vi "MyRIO_Main.vi"() -> ()   [LabVIEW 2019]
uses:
  <vilib>/myRIO/Instrument Drivers/Onboard IO/DIO/typedefs/DIO Reference.ctl
  <vilib>/myRIO/Common/Instrument Driver Framework/Utilities/typedefs/myRIO Generic Hardware Reference.ctl
  <vilib>/myRIO/Common/Instrument Driver Framework/Utilities/typedefs/Hardware Version Enum.ctl
  <vilib>/myRIO/Common/Instrument Driver Framework/Utilities/typedefs/myRIO v1.0 Reference.ctl
  <vilib>/myRIO/Common/Instrument Driver Framework/Utilities/typedefs/Generic FPGA Reference.ctl
  <vilib>/myRIO/Common/Instrument Driver Framework/myRIO v1.0/DIO/typedefs/DIO Channels List.ctl
  <vilib>/myRIO/Common/Instrument Driver Framework/myRIO v1.0/DIO/typedefs/DIO Channels Enum.ctl
  <vilib>/userDefined/High Color/nirio_resource_hc.ctl
  <vilib>/myRIO/Instrument Drivers/Onboard Devices/Accelerometer/typedefs/Accelerometer Reference.ctl
  <vilib>/myRIO/Common/Instrument Driver Framework/myRIO v1.0/Accelerometer/typedefs/Accelerometer Channels List.ctl
  <vilib>/myRIO/Common/Instrument Driver Framework/myRIO v1.0/Accelerometer/typedefs/Accelerometer Channels Enum.ctl
  <vilib>/myRIO/Common/Instrument Driver Framework/Utilities/vis/Is FPGA Ref Available.vi
  <vilib>/myRIO/Common/Instrument Driver Framework/myRIO v1.0/DIO/vis/myRIO v1.1 Open DIO.vi
  <vilib>/myRIO/Instrument Drivers/Onboard IO/DIO/vis/Read.vi
  <vilib>/myRIO/Common/Instrument Driver Framework/myRIO v1.0/Accelerometer/vis/myRIO v1.1 Open Accelerometer.vi
  <vilib>/myRIO/Instrument Drivers/Onboard Devices/Accelerometer/vis/Read.vi
  <vilib>/myRIO/Instrument Drivers/Onboard IO/DIO/vis/Write.vi
  <vilib>/myRIO/Common/Instrument Driver Framework/Utilities/vis/Validate Channels.vi
  <vilib>/myRIO/Common/Instrument Driver Framework/myRIO v1.0/DIO/vis/myRIO v1.0 Reserve DIO.vi
  <vilib>/myRIO/Common/Instrument Driver Framework/myRIO v1.0/Accelerometer/vis/myRIO v1.0 Reserve Accelerometer.vi
  <vilib>/myRIO/Common/Instrument Driver Framework/myRIO v1.0/Resource Manager/vis/myRIO v1.0 Reserve Channel List.vi
  <vilib>/myRIO/Common/Instrument Driver Framework/myRIO v1.0/DIO/vis/myRIO v1.0 Build MUX Configuration DIO.vi
  <vilib>/myRIO/Common/Instrument Driver Framework/myRIO v1.0/Accelerometer/vis/myRIO v1.0 Build MUX Configuration Accelerometer.vi
  <vilib>/myRIO/Common/Instrument Driver Framework/myRIO v1.0/Resource Manager/vis/myRIO v1.0 Reserve Channel.vi
  <vilib>/myRIO/Common/Instrument Driver Framework/myRIO v1.0/Resource Manager/vis/myRIO v1.0 Unreserve Channel.vi
  <vilib>/myRIO/Common/Instrument Driver Framework/myRIO v1.0/Resource Manager/vis/myRIO v1.0 Create Configuration List.vi
  <vilib>/myRIO/Common/Instrument Driver Framework/myRIO v1.0/Resource Manager/vis/myRIO v1.0 Build Mutex Name.vi
  <vilib>/Utility/VariantDataType/GetNumericInfo.vi
  <vilib>/Utility/error.llb/Error Cluster From Error Code.vi
  <vilib>/myRIO/Common/Instrument Driver Framework/myRIO v1.0/myRIO v1.1 Open.vi
  <vilib>/myRIO/Common/Instrument Driver Framework/Utilities/vis/IO Manager.vi
  <vilib>/myRIO/Common/Instrument Driver Framework/Utilities/vis/Configuration Manager.vi
  <vilib>/myRIO/Common/Instrument Driver Framework/myRIO v1.0/Resource Manager/vis/myRIO v1.0 Configure IO.vi
  <vilib>/myRIO/Common/Instrument Driver Framework/myRIO v1.0/myRIO v1.0 Close.vi
  <vilib>/myRIO/Common/Instrument Driver Framework/myRIO v1.0/DIO/vis/myRIO v1.0 Read DIO.vi
  <vilib>/myRIO/Common/Instrument Driver Framework/myRIO v1.0/Accelerometer/vis/myRIO v1.0 Get Scaling Constant Accelerometer.vi
  <vilib>/myRIO/Common/Instrument Driver Framework/myRIO v1.0/Accelerometer/vis/myRIO v1.0 Read Accelerometer.vi
  <vilib>/myRIO/Common/Instrument Driver Framework/myRIO v1.0/DIO/vis/myRIO v1.0 Write DIO.vi
  <vilib>/myRIO/Express VI/Onboard Devices/Button/Button Express VI.xnode
  <vilib>/myRIO/Instrument Drivers/Onboard IO/DIO/vis/myRIO DIO Open.xnode
  <vilib>/myRIO/Express VI/Onboard Devices/Accelerometer/Accelerometer Express VI.xnode
  <vilib>/myRIO/Instrument Drivers/Onboard Devices/Accelerometer/vis/myRIO Accelerometer Open.xnode
  <vilib>/myRIO/Express VI/Onboard Devices/LED/LED Express VI.xnode
  <vilib>/myRIO/Instrument Drivers/Onboard IO/DIO/DIO.lvlib
  <vilib>/myRIO/Instrument Drivers/Onboard Devices/Accelerometer/Accelerometer.lvlib
panel:
  out "angke":dbl
  out "z":dbl
  out "y":dbl
  in  "stop":bool
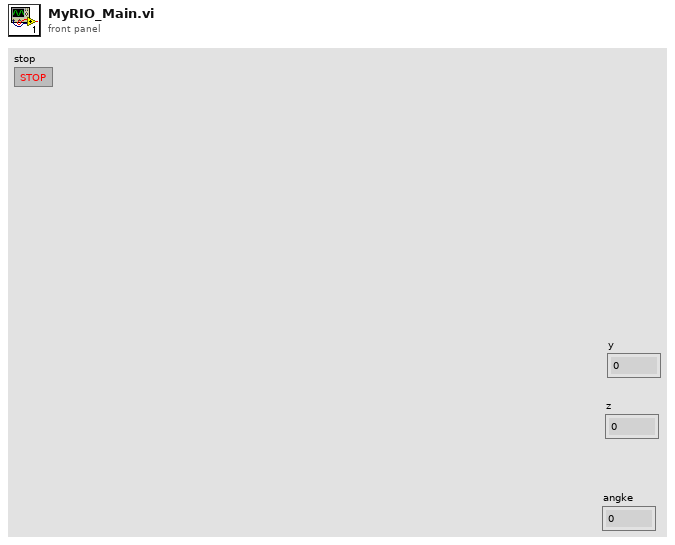
[diagram p1: front panel]
types:
  T1 = typedef "Accelerometer.lvlib/Accelerometer Reference.ctl" = cluster{"myRIO Reference":T2, "Accelerometer Channels List":T6, "LSB Weight":dbl}
  T2 = typedef "myRIO Generic Hardware Reference.ctl" = cluster{"myRIO Model":T3, "myRIO Hardware Reference":T4}
  T3 = typedef "Hardware Version Enum.ctl" = enum16{"Unknown", "myRIO-1900", "myRIO-1950", "roboRIO", "NI ELVIS RIO CM", "ELVIS III"}
  T4 = typedef "myRIO v1.0 Reference.ctl" = cluster{"Generic FPGA Reference":T5, "Allow multiple opens":bool}
  T5 = typedef "Generic FPGA Reference.ctl" = refnum<k20>
  T6 = typedef "Accelerometer Channels List.ctl" = T7[]
  T7 = typedef "Accelerometer Channels Enum.ctl" = enum16{"Not Connected", "X-Axis", "Y-Axis", "Z-Axis"}
  T8 = typedef "nirio_resource_hc.ctl" = tag
  T9 = typedef "DIO.lvlib/DIO Reference.ctl" = cluster{"myRIO Reference":T2, "DIO Channels List":T10}
  T10 = typedef "DIO Channels List.ctl" = T11[]
  T11 = typedef "DIO Channels Enum.ctl" = enum16{"Not Connected", "C/DIO0", "C/DIO1", "C/DIO2", "C/DIO3", "C/DIO4", "C/DIO5", "C/DIO6", "C/DIO7", "A/DIO0", "A/DIO1", "A/DIO2", "A/DIO3", "A/DIO4", "A/DIO5", "A/DIO6", "A/DIO7", "A/DIO8", "A/DIO9", "A/DIO10", "A/DIO11", "A/DIO12", "A/DIO13", "A/DIO14", "A/DIO15", "A/DIO16", "A/DIO17", "A/DIO18", "A/DIO19", "B/DIO0", "B/DIO1", "B/DIO2", "B/DIO3", "B/DIO4", "B/DIO5", "B/DIO6", "B/DIO7", "B/DIO8", "B/DIO9", "B/DIO10", "B/DIO11", "B/DIO12", "B/DIO13", "B/DIO14", "B/DIO15", "B/DIO16", "B/DIO17", "B/DIO18", "B/DIO19", "LED0", "LED1", "LED2", "LED3", "Button0", "DIO/DIO0", "DIO/DIO1", "DIO/DIO2", "DIO/DIO3", "DIO/DIO4", "DIO/DIO5", "DIO/DIO6", "DIO/DIO7", "DIO/DIO8", "DIO/DIO9", "SPI/CS0", "SPI/CS1", "SPI/CS2", "SPI/CS3", "LED RADIO (Green)", "LED RADIO (Red)", "LED COMM (Green)", "LED COMM (Red)", "LED MODE (Green)", "LED MODE (Red)"}
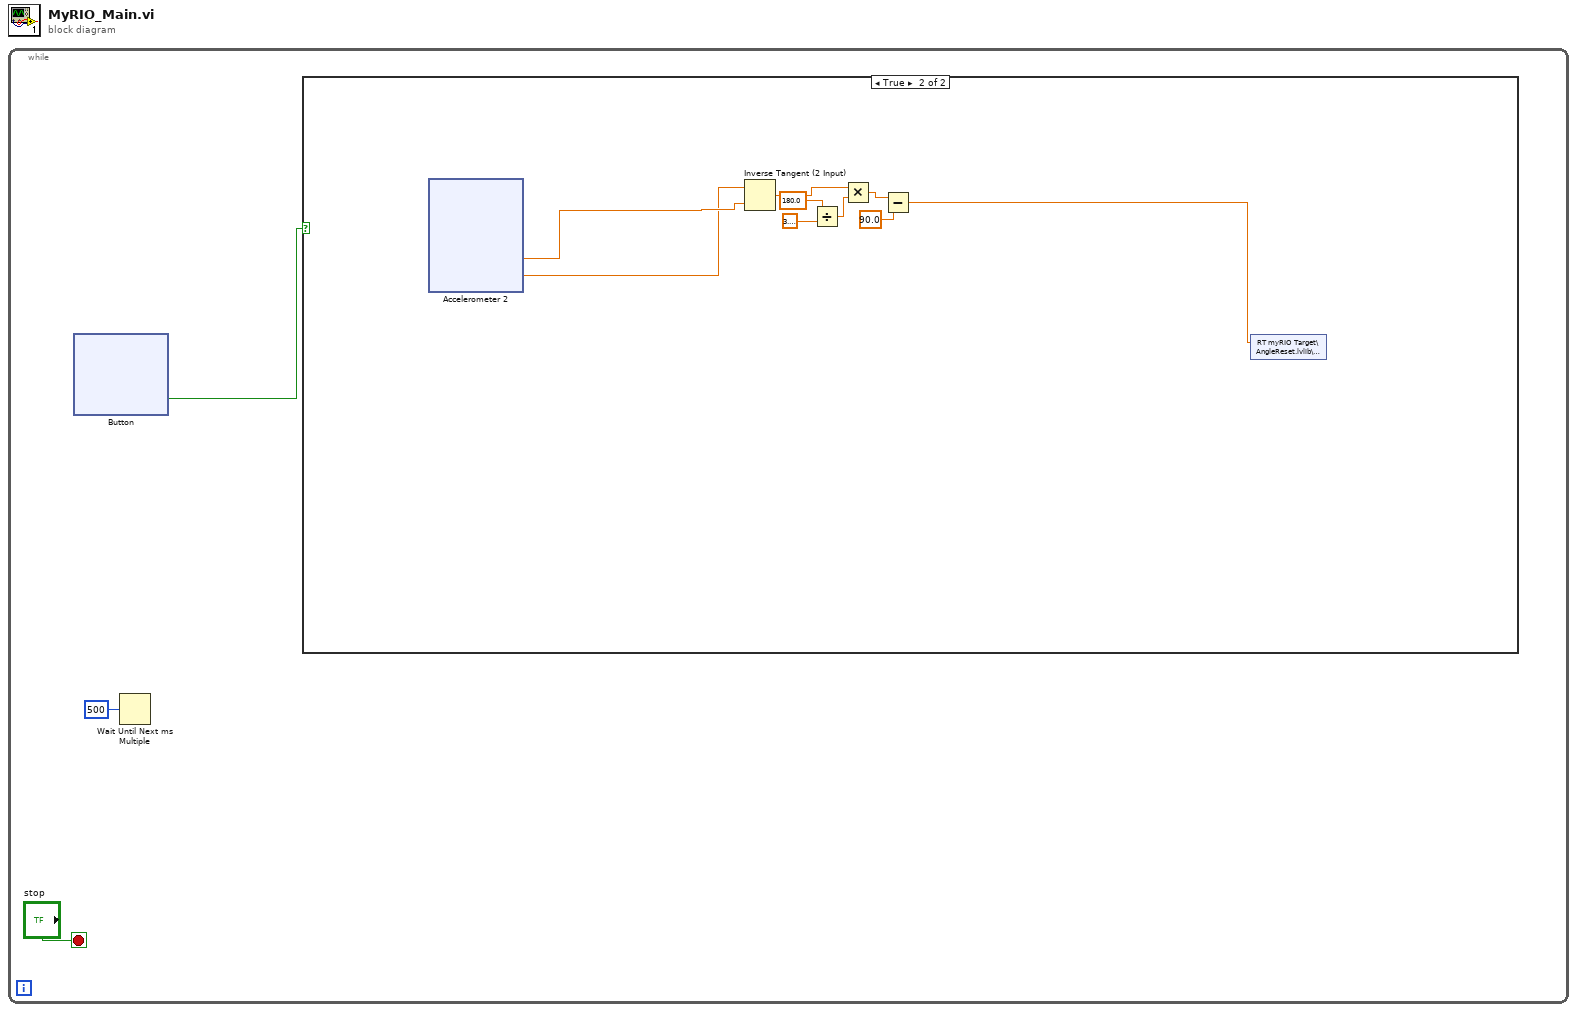
[diagram p0: block diagram]
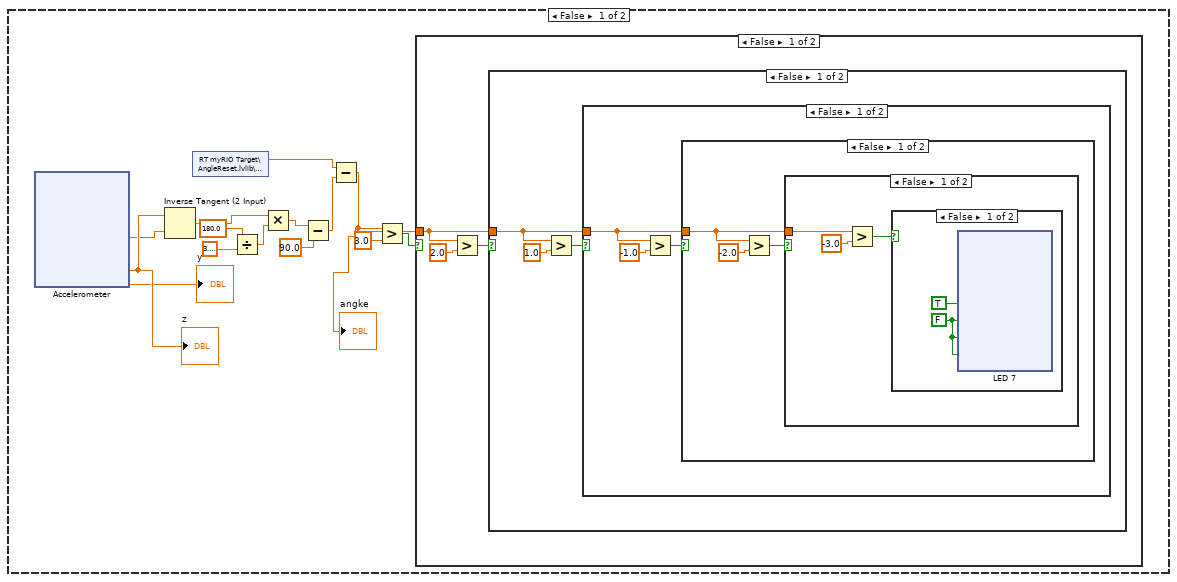
[diagram p2: hidden frame]
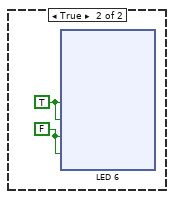
[diagram p3: hidden frame]
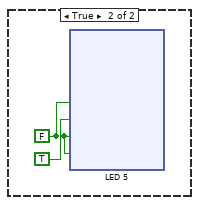
[diagram p4: hidden frame]
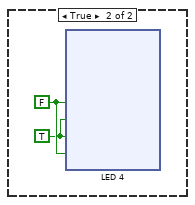
[diagram p5: hidden frame]
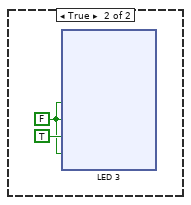
[diagram p6: hidden frame]
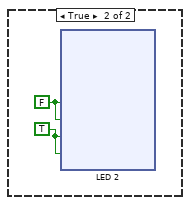
[diagram p7: hidden frame]
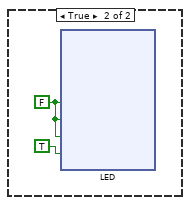
[diagram p8: hidden frame]
diagram:
  n1 = while {
    stop <- "stop" stop-if-true
    n2 = xnode "Button"() -> ("Value"=w1:bool)  [unwired: 1 in, 1 out]
    n3 = Wait Until Next ms Multiple(millisecond multiple=u32 500) -> ()  [unwired: 1 out]
    n4 = case shown="True" w1 {
      frame False {
        n5 = xnode "Accelerometer"() -> ("Y-Axis"=w14:dbl, "Z-Axis"=w15:dbl)  [unwired: 1 in, 2 out]
        "z" <- w15
        "y" <- w14
        n6 = Inverse Tangent (2 Input)(1:w14, 2:w15) -> (0:w12:dbl)
        n7 = shared-variable "RT myRIO Target\\AngleReset.lvlib\\Angle"() -> (w6:dbl)  [unwired: 1 in, 1 out]
        n8 = Divide(x=180.0, y=3.141592653589793) -> (x/y=w11:dbl)
        n9 = Multiply(x=w12, y=w11) -> (x*y=w16:dbl)
        n10 = Subtract(x=w16, y=90.0) -> (x-y=w5:dbl)
        n11 = Subtract(x=w6, y=w5) -> (x-y=w4:dbl)
        "angke" <- w4
        n12 = Greater?(x=w4, y=3.0) -> (0:w13:bool)
        n13 = case shown="False" w13 {
          tunnel: w4 -> [w56 _]
          frame False {
            n14 = Greater?(x=w56, y=2.0) -> (0:w58:bool)
            n15 = case shown="False" w58 {
              tunnel: w56 -> [w59 _]
              frame False {
                n16 = Greater?(x=w59, y=1.0) -> (0:w60:bool)
                n17 = case shown="False" w60 {
                  tunnel: w59 -> [w62 _]
                  frame False {
                    n18 = Greater?(x=w62, y=-1.0) -> (0:w63:bool)
                    n19 = case shown="False" w63 {
                      tunnel: w62 -> [w65 _]
                      frame False {
                        n20 = Greater?(x=w65, y=-2.0) -> (0:w67:bool)
                        n21 = case shown="False" w67 {
                          tunnel: w65 -> [w68 _]
                          frame False {
                            n22 = Greater?(x=w68, y=-3.0) -> (0:w69:bool)
                            n23 = case shown="False" w69 {
                              frame False {
                                w71 = FALSE
                                n24 = xnode "LED 7"("LED0"=TRUE, "LED1"=w71, "LED2"=w71, "LED3"=w71) -> ()  [unwired: 1 in, 1 out]
                              }
                              frame True {
                                w112 = TRUE
                                w111 = FALSE
                                n25 = xnode "LED 6"("LED0"=w112, "LED1"=w112, "LED2"=w111, "LED3"=w111) -> ()  [unwired: 1 in, 1 out]
                              }
                            }
                          }
                          frame True {
                            w151 = FALSE
                            n26 = xnode "LED 5"("LED0"=w151, "LED1"=TRUE, "LED2"=w151, "LED3"=w151) -> ()  [unwired: 1 in, 1 out]
                          }
                        }
                      }
                      frame True {
                        w191 = TRUE
                        w192 = FALSE
                        n27 = xnode "LED 4"("LED0"=w192, "LED1"=w191, "LED2"=w191, "LED3"=w192) -> ()  [unwired: 1 in, 1 out]
                      }
                    }
                  }
                  frame True {
                    w231 = FALSE
                    n28 = xnode "LED 3"("LED0"=w231, "LED1"=w231, "LED2"=TRUE, "LED3"=w231) -> ()  [unwired: 1 in, 1 out]
                  }
                }
              }
              frame True {
                w271 = TRUE
                w272 = FALSE
                n29 = xnode "LED 2"("LED0"=w272, "LED1"=w272, "LED2"=w271, "LED3"=w271) -> ()  [unwired: 1 in, 1 out]
              }
            }
          }
          frame True {
            w312 = FALSE
            n30 = xnode "LED"("LED0"=w312, "LED1"=w312, "LED2"=w312, "LED3"=TRUE) -> ()  [unwired: 1 in, 1 out]
          }
        }
      }
      frame True {
        n31 = xnode "Accelerometer 2"() -> ("X-Axis"=w353:dbl, "Z-Axis"=w352:dbl)  [unwired: 1 in, 1 out]
        n32 = Inverse Tangent (2 Input)(1:w353, 2:w352) -> (0:w358:dbl)
        n33 = Divide(x=180.0, y=3.141592653589793) -> (x/y=w357:dbl)
        n34 = Multiply(x=w358, y=w357) -> (x*y=w359:dbl)
        n35 = Subtract(x=w359, y=90.0) -> (x-y=w351:dbl)
        n36 = shared-variable "RT myRIO Target\\AngleReset.lvlib\\Angle"(w351) -> ()  [unwired: 1 in, 1 out]
      }
    }
  }
